vi "开机添加默认配置文件.vi"(8 "error in (no error)":errorcluster caption="错误输入（无错误）", 11 "恢复默认方式":enum16{"无配置开机恢复", "手动恢复"}(ring)) -> (0 "error out":errorcluster caption="错误输出")   [LabVIEW 2016, in "环境动力监测库.lvlib"]
uses:
  <vilib>/Utility/config.llb/NI_LVConfig.lvlib
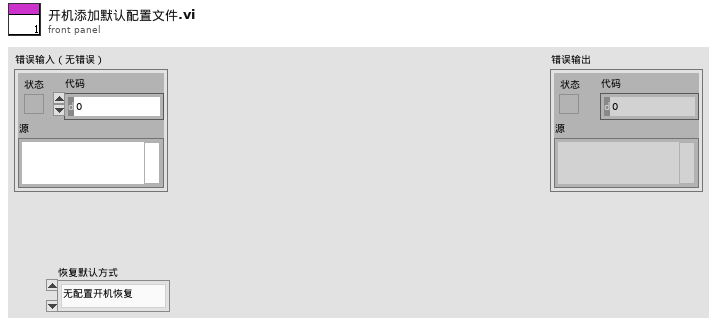
[diagram p1: front panel]
types:
  T1 = typedef "NI_LVConfig.lvlib/Config Data RefNum.ctl" = refnum<k1>
  T2 = cluster{"监测项描述:输出":string, "连接方式":enum16{"串口", "TCP"}, "端口":string, "IP address:":string, "Port:":string, "站号":u64, "传感器型号":string, "波特率":u64, "data bits":u64, "停止位":u16, "奇偶校验":u16}
  T3 = cluster{"监测项描述:输出":string, "端口":enum16{"AI0", "AI1", "AI2", "AI3", "AI4", "DI0", "DI1", "DI2", "DI3", "DI4", "DO0", "DO1", "DO2", "DO3", "DO4", "X0", "X1", "X2", "X3", "X4", "X5", "X6", "X7", "X8", "X9"}, "告警方式":enum32{"禁用告警", "闭合告警", "断开告警"}, "传感器型号":enum16{"PLC", "ZLAN"}}
  T4 = cluster{"监测项描述:输出":string, "端口":enum16{"AI0", "AI1", "AI2", "AI3", "AI4", "DI0", "DI1", "DI2", "DI3", "DI4", "DO0", "DO1", "DO2", "DO3", "DO4", "X0", "X1", "X2", "X3", "X4", "X5", "X6", "X7", "X8", "X9"}, "告警方式":enum32{"禁用告警", "闭合告警", "断开告警"}, "传感器型号":enum16{"PLC", "ZLAN"}, "声光告警启用":bool}
  T5 = cluster{"监测项描述:输出":string, "端口":enum16{"AI0", "AI1", "AI2", "AI3", "AI4", "DI0", "DI1", "DI2", "DI3", "DI4", "DO0", "DO1", "DO2", "DO3", "DO4", "X0", "X1", "X2", "X3", "X4", "X5", "X6", "X7", "X8", "X9"}, "告警方式":enum32{"禁用告警", "闭合告警", "断开告警"}, "传感器型号":enum16{"PLC", "ZLAN", "ART"}, "声光告警启用":bool}
  T6 = enum16{"AI0", "AI1", "AI2", "AI3", "AI4", "DI0", "DI1", "DI2", "DI3", "DI4", "DO0", "DO1", "DO2", "DO3", "DO4", "X0", "X1", "X2", "X3", "X4", "X5", "X6", "X7", "X8", "X9"}[]
  T7 = cluster{"漏水监测配置":cluster{"监测项描述:输出":string, "端口:":enum16{"AI0", "AI1", "AI2", "AI3", "AI4", "DI0", "DI1", "DI2", "DI3", "DI4", "DO0", "DO1", "DO2", "DO3", "DO4", "X0", "X1", "X2", "X3", "X4", "X5", "X6", "X7", "X8", "X9", "X10", "X11", "X12", "X13", "X14", "X15", "X16", "X17", "X18", "X19", "X20", "X21", "X22", "X23"}, "告警参数:":enum32{"禁用告警", "闭合告警", "断开告警"}, "传感器型号:":enum16{"PLC", "ZLAN", "ART"}, "声光告警启用":bool}, "门禁开关监测配置":cluster{"监测项描述:输出":string, "端口:":enum16{"AI0", "AI1", "AI2", "AI3", "AI4", "DI0", "DI1", "DI2", "DI3", "DI4", "DO0", "DO1", "DO2", "DO3", "DO4", "X0", "X1", "X2", "X3", "X4", "X5", "X6", "X7", "X8", "X9", "X10", "X11", "X12", "X13", "X14", "X15", "X16", "X17", "X18", "X19", "X20", "X21", "X22", "X23"}, "告警参数:":enum32{"禁用告警", "闭合告警", "断开告警"}, "传感器型号:":enum16{"PLC", "ZLAN", "ART"}, "声光告警启用":bool}, "门禁开关监测配置2":cluster{"监测项描述:输出":string, "端口:":enum16{"AI0", "AI1", "AI2", "AI3", "AI4", "DI0", "DI1", "DI2", "DI3", "DI4", "DO0", "DO1", "DO2", "DO3", "DO4", "X0", "X1", "X2", "X3", "X4", "X5", "X6", "X7", "X8", "X9", "X10", "X11", "X12", "X13", "X14", "X15", "X16", "X17", "X18", "X19", "X20", "X21", "X22", "X23"}, "告警参数:":enum32{"禁用告警", "闭合告警", "断开告警"}, "传感器型号:":enum16{"PLC", "ZLAN", "ART"}, "声光告警启用":bool}, "温湿度监测配置":cluster{"监测项描述:输出":string, "端口:":enum16{"AI0", "AI1", "AI2", "AI3", "AI4", "DI0", "DI1", "DI2", "DI3", "DI4", "DO0", "DO1", "DO2", "DO3", "DO4", "X0", "X1", "X2", "X3", "X4", "X5", "X6", "X7", "X8", "X9", "X10", "X11", "X12", "X13", "X14", "X15", "X16", "X17", "X18", "X19", "X20", "X21", "X22", "X23"}, "告警参数:":enum32{"禁用告警", "闭合告警", "断开告警"}, "传感器型号:":enum16{"PLC", "ZLAN", "ART"}, "声光告警启用":bool}, "烟雾监测配置":cluster{"监测项描述:输出":string, "端口:":enum16{"AI0", "AI1", "AI2", "AI3", "AI4", "DI0", "DI1", "DI2", "DI3", "DI4", "DO0", "DO1", "DO2", "DO3", "DO4", "X0", "X1", "X2", "X3", "X4", "X5", "X6", "X7", "X8", "X9", "X10", "X11", "X12", "X13", "X14", "X15", "X16", "X17", "X18", "X19", "X20", "X21", "X22", "X23"}, "告警参数:":enum32{"禁用告警", "闭合告警", "断开告警"}, "传感器型号:":enum16{"PLC", "ZLAN", "ART"}, "声光告警启用":bool}, "冰箱监测配置":cluster{"监测项描述:输出":string, "端口:":enum16{"AI0", "AI1", "AI2", "AI3", "AI4", "DI0", "DI1", "DI2", "DI3", "DI4", "DO0", "DO1", "DO2", "DO3", "DO4", "X0", "X1", "X2", "X3", "X4", "X5", "X6", "X7", "X8", "X9", "X10", "X11", "X12", "X13", "X14", "X15", "X16", "X17", "X18", "X19", "X20", "X21", "X22", "X23"}, "告警参数:":enum32{"禁用告警", "闭合告警", "断开告警"}, "传感器型号:":enum16{"PLC", "ZLAN", "ART"}, "声光告警启用":bool}, "排气扇监测配置":cluster{"监测项描述:输出":string, "端口:":enum16{"AI0", "AI1", "AI2", "AI3", "AI4", "DI0", "DI1", "DI2", "DI3", "DI4", "DO0", "DO1", "DO2", "DO3", "DO4", "X0", "X1", "X2", "X3", "X4", "X5", "X6", "X7", "X8", "X9", "X10", "X11", "X12", "X13", "X14", "X15", "X16", "X17", "X18", "X19", "X20", "X21", "X22", "X23"}, "告警参数:":enum32{"禁用告警", "闭合告警", "断开告警"}, "传感器型号:":enum16{"PLC", "ZLAN", "ART"}, "声光告警启用":bool}, "红外入侵监测配置":cluster{"监测项描述:输出":string, "端口:":enum16{"AI0", "AI1", "AI2", "AI3", "AI4", "DI0", "DI1", "DI2", "DI3", "DI4", "DO0", "DO1", "DO2", "DO3", "DO4", "X0", "X1", "X2", "X3", "X4", "X5", "X6", "X7", "X8", "X9", "X10", "X11", "X12", "X13", "X14", "X15", "X16", "X17", "X18", "X19", "X20", "X21", "X22", "X23"}, "告警参数:":enum32{"禁用告警", "闭合告警", "断开告警"}, "传感器型号:":enum16{"PLC", "ZLAN", "ART"}, "声光告警启用":bool}, "振动监测配置":cluster{"监测项描述:输出":string, "端口:":enum16{"AI0", "AI1", "AI2", "AI3", "AI4", "DI0", "DI1", "DI2", "DI3", "DI4", "DO0", "DO1", "DO2", "DO3", "DO4", "X0", "X1", "X2", "X3", "X4", "X5", "X6", "X7", "X8", "X9", "X10", "X11", "X12", "X13", "X14", "X15", "X16", "X17", "X18", "X19", "X20", "X21", "X22", "X23"}, "告警参数:":enum32{"禁用告警", "闭合告警", "断开告警"}, "传感器型号:":enum16{"PLC", "ZLAN", "ART"}, "声光告警启用":bool}}
  T8 = cluster{"市电监测":bool, "用水量监测":bool, "烟雾监测":bool, "温度湿度":bool, "振动监测":bool, "红外入侵监测":bool, "漏水监测":bool, "门禁开关监测":bool, "门禁开关监测2":bool, "视频监测":bool, "UPS监测":bool, "空调监测":bool, "冰箱监测":bool, "排气扇监测":bool, "蓄电池监测":bool, "蓄电池监测2":bool, "GPS监测":bool, "北斗监测":bool, "气象监测":bool, "智能门禁监测":bool}
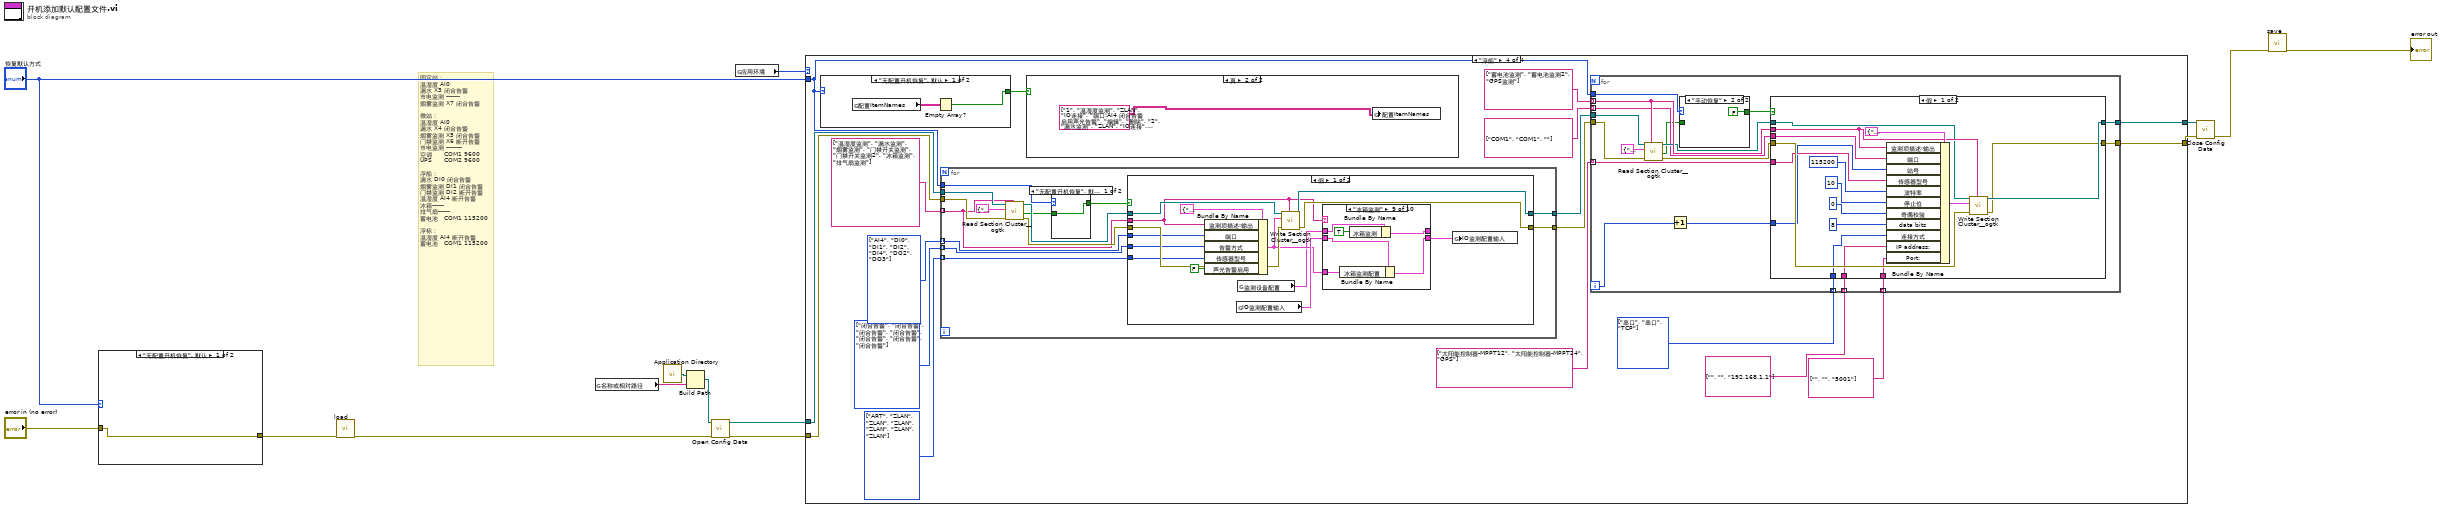
[diagram p0: block diagram]
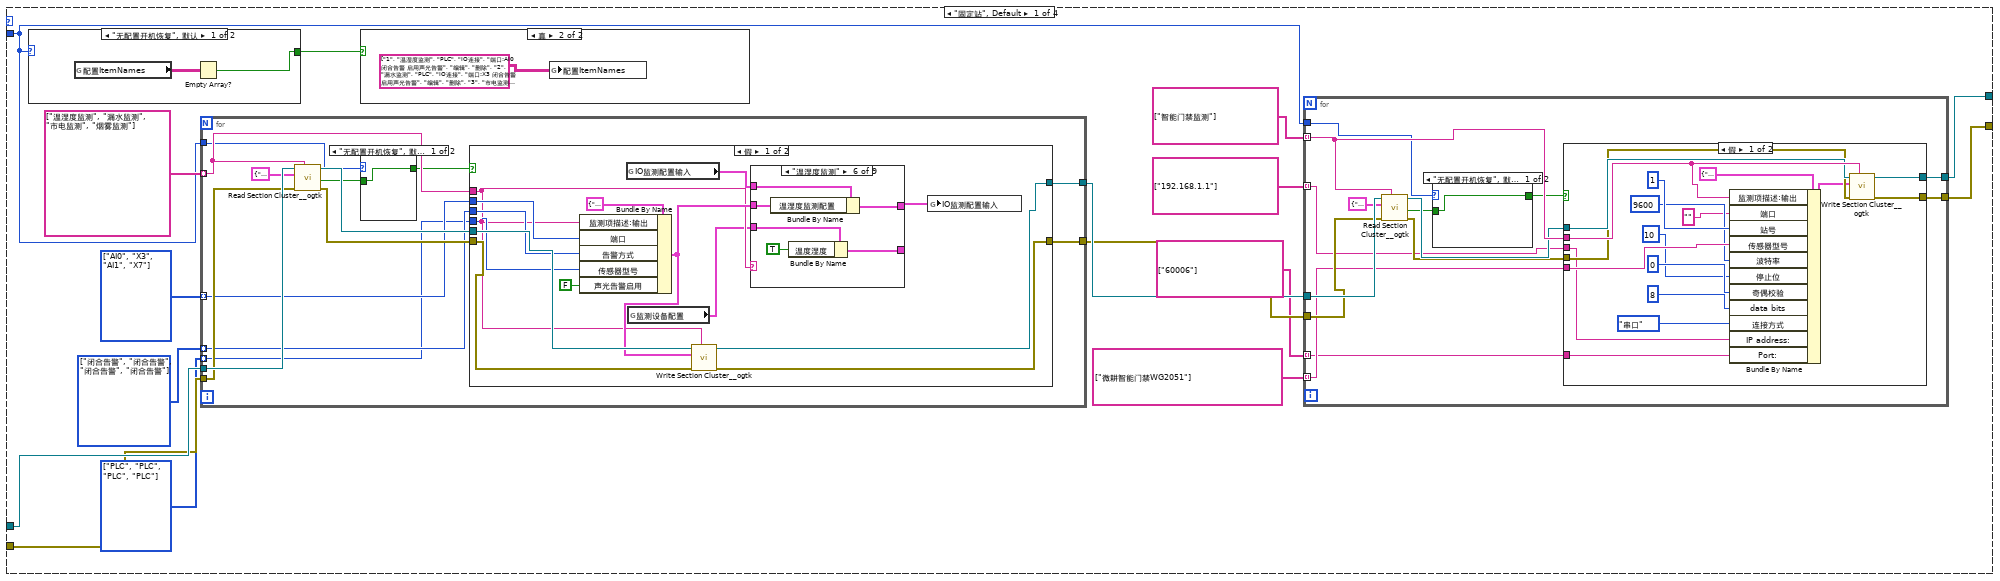
[diagram p3: hidden frame]
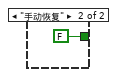
[diagram p4: hidden frame]
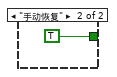
[diagram p6: hidden frame]
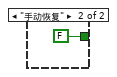
[diagram p8: hidden frame]
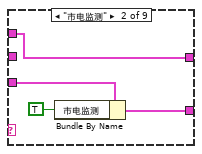
[diagram p10: hidden frame]
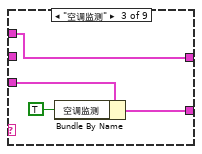
[diagram p11: hidden frame]
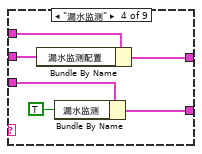
[diagram p12: hidden frame]
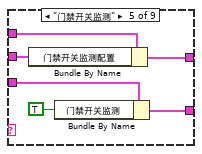
[diagram p13: hidden frame]
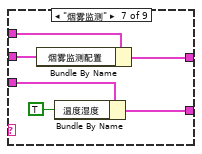
[diagram p14: hidden frame]
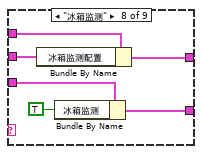
[diagram p15: hidden frame]
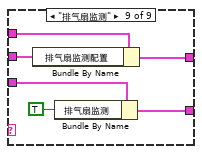
[diagram p16: hidden frame]
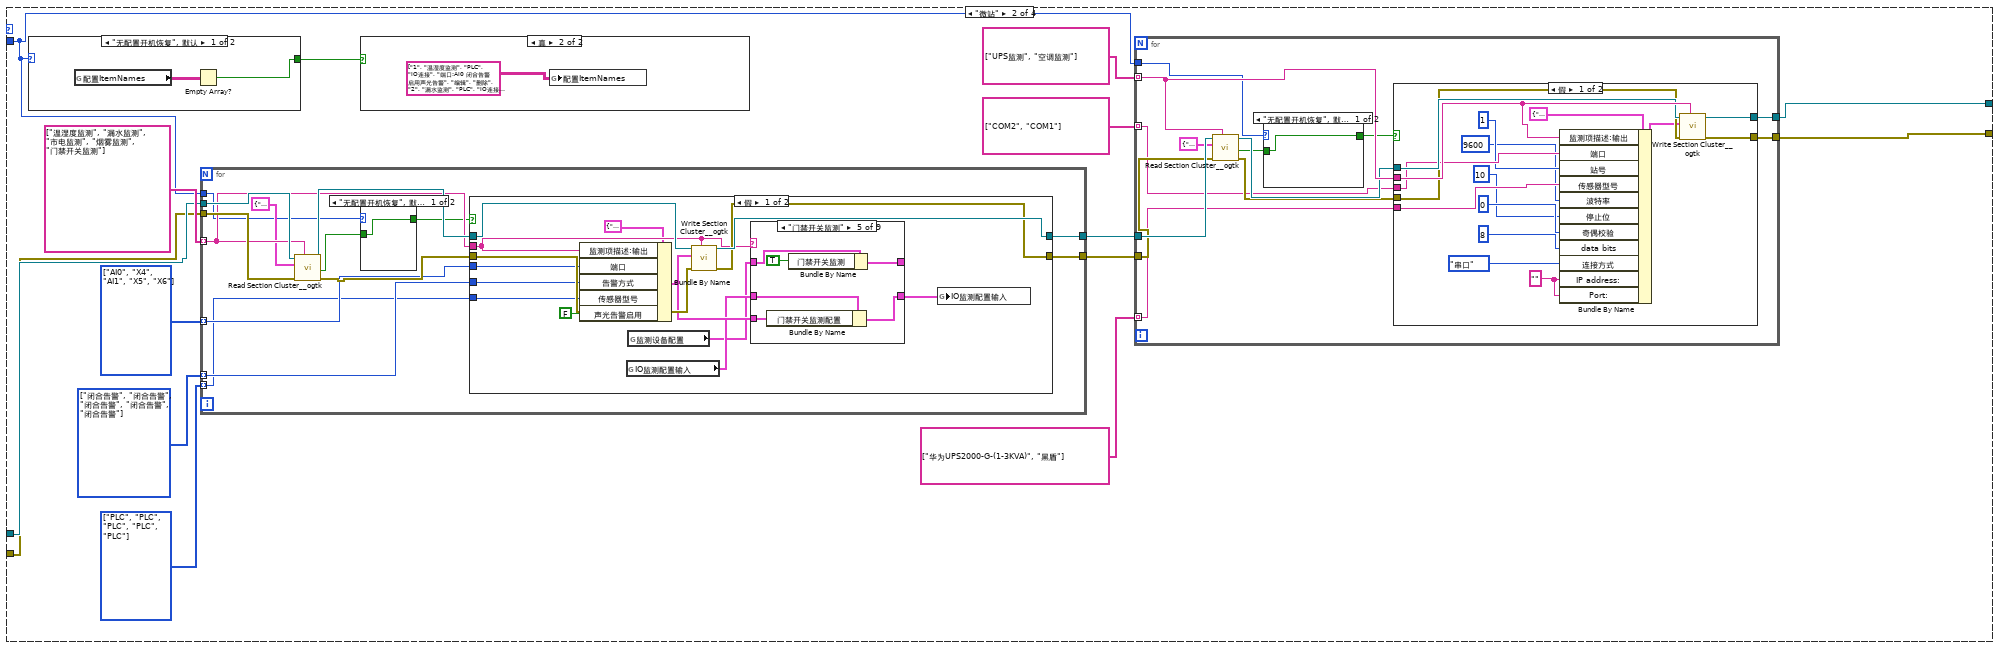
[diagram p18: hidden frame]
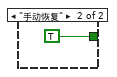
[diagram p19: hidden frame]
diagram:
  # "固定站：\n温湿度 AI0\n漏水 X3 闭合告警\n市电监测 -------\n烟雾监测 X7 闭合告警\n\n微站：\n温湿度 AI0\n漏水 X4 闭合告警\n烟雾监测 X5 闭合告警\n门禁监测 X6 断开告警\n市电监测 --------\n空调      COM1 9600\nUPS      COM2 9600\n\n浮船：\n漏水 DI0 闭合告警\n烟雾监测 DI1 闭合告警\n门禁监测 DI2 断开告警\n温湿度 AI4 断开告警\n冰箱------\n排气扇------\n蓄电池   COM1 115200\n\n浮标：\n温湿度 AI4 断开告警\n蓄电池   COM1 115200"
  n1 = case shown="\"无配置开机恢复\", 默认" "恢复默认方式" {
    tunnel: "error in (no error)" -> [w15 w16]
    tunnel: [w15 w16] -> w3
    frame "无配置开机恢复", Default {
    }
    frame "手动恢复" {
    }
  }
  n2 = call "load.vi"("error in (no error)"=w3) -> ("error out"=w7:errorcluster)  [unwired: 10 in]
  n3 = global read "内部交互全局变量.vi" "名称或相对路径"() -> (w4:string)
  n4 = call <vilib>:"Application Directory.vi"() -> ("Application Directory"=w13:path)
  n5 = Build Path(base path=w13, name or relative path=w4) -> (appended path=w12:path)
  n6 = call <vilib>:"Open Config Data.vi"("error in (no error)"=w7, "configuration file path"=w12) -> ("error out"=w10:errorcluster, "refnum"=w11:T1)  [unwired: 7 in, 1 out]
  n7 = global read "外部交互全局变量.vi" "应用环境"() -> (w14:enum16{"固定站", "微站", "浮标", "浮船"})
  n8 = case shown="\"浮船\"" w14 {
    tunnel: w11 -> [w31 w163 w293 w426]
    tunnel: w10 -> [w30 w162 w292 w425]
    tunnel: [w19 w158 w288 w421] -> w9
    tunnel: [w18 w157 w287 w420] -> w8
    tunnel: "恢复默认方式" -> [w20 w150 w280 w413]
    frame "固定站", Default {
      w27 = enum16{"PLC", "ZLAN"}[] [enum."PLC", enum."PLC", enum."PLC", enum."PLC"] items=["PLC", "ZLAN"]
      w28 = enum32{"禁用告警", "闭合告警", "断开告警"}[] [enum."闭合告警", enum."闭合告警", enum."闭合告警", enum."闭合告警"] items=["禁用告警", "闭合告警", "断开告警"]
      w29 = T6 [enum."AI0", enum."X3", enum."AI1", enum."X7"] items=["AI0", "AI1", "AI2", "AI3", "AI4", "DI0", "DI1", "DI2", "DI3", "DI4", "DO0", "DO1", "DO2", "DO3", "DO4", "X0", "X1", "X2", "X3", "X4", "X5", "X6", "X7", "X8", "X9"]
      n9 = case shown="\"无配置开机恢复\", 默认" w20 {
        tunnel: [w68 TRUE ("empty?")] -> w26
        frame "无配置开机恢复", Default {
          n10 = global read "断电保存全局变量.vi" "配置ItemNames"() -> (w69:string[][])
          n11 = Empty Array?(array=w69) -> (empty?=w68:bool)
        }
        frame "手动恢复" {
        }
      }
      n12 = for {
        tunnel: string[] ["温湿度监测", "漏水监测", "市电监测", "烟雾监测"] -> [w81] mode=indexing
        tunnel: w31 -> [w85]
        tunnel: w30 -> [w84]
        tunnel: w29 -> [w80] mode=indexing
        tunnel: w28 -> [w79] mode=indexing
        tunnel: w27 -> [w78] mode=indexing
        tunnel: [w77] -> w22
        tunnel: [w76] -> w21
        tunnel: w20 -> [w72]
        n13 = call <userlib>:"Read Section Cluster__ogtk.vi"("section (optional)"=w81, "error in (no error)"=w84, "Section Formatted Cluster Type"=T3 {"监测项描述:输出"="烟雾监测", "端口"=enum."X8", "告警方式"=enum."闭合告警", "传感器型号"=enum."PLC"} ("簇1输入"), "refnum"=w85) -> ("error out"=w82:errorcluster, "all found?"=w74:bool, "dup refnum"=w83:T1)  [unwired: 3 in, 2 out]
        n14 = case shown="\"无配置开机恢复\", 默认" w72 {
          tunnel: [w86 FALSE] -> w73
          tunnel: w74 -> [w86 _]
          frame "无配置开机恢复", Default {
          }
          frame "手动恢复" {
          }
        }
        n15 = case shown="假" w73 {
          tunnel: w83 -> [w101 w149]
          tunnel: w82 -> [w100 w148]
          tunnel: w81 -> [w92 _]
          tunnel: w80 -> [w99 _]
          tunnel: w79 -> [w94 _]
          tunnel: w78 -> [w98 _]
          tunnel: [w97 w149] -> w77
          tunnel: [w96 w148] -> w76
          frame False {
            n16 = Bundle By Name(cluster=T4 {"监测项描述:输出"="", "端口"=enum."AI0", "告警方式"=enum."禁用告警", "传感器型号"=enum."PLC", "声光告警启用"=FALSE} ("簇1输出"), "监测项描述:输出"=w92, "端口"=w99, "告警方式"=w94, "传感器型号"=w98, "声光告警启用"=FALSE) -> (w93:T4)
            n17 = global read "断电保存全局变量.vi" "IO监测配置输入"() -> (w95:T7)
            n18 = global read "断电保存全局变量.vi" "监测设备配置"() -> (w91:T8)
            n19 = call <userlib>:"Write Section Cluster__ogtk.vi"("section (optional)"=w92, "error in (no error)"=w100, "Section Formatted Cluster"=w93, "refnum"=w101) -> ("error out"=w96:errorcluster, "dup refnum"=w97:T1)  [unwired: 6 in]
            n20 = case shown="\"温湿度监测\"" w92 {
              tunnel: w95 -> [w103 w107 w111 w117 w123 w129 w135 w141 w147]
              tunnel: [w103 w107 w111 w116 w122 w128 w134 w140 w146] -> w90
              tunnel: w93 -> [_ _ _ w115 w121 w127 w133 w139 w145]
              tunnel: w91 -> [w102 w106 w110 w114 w119 w126 w132 w138 w144]
              tunnel: [w102 w104 w109 w113 w120 w125 w131 w137 w143] -> _
              frame "假", Default {
              }
              frame "市电监测" {
                n21 = Bundle By Name(cluster=w106, "市电监测"=TRUE) -> (w104:T8)
              }
              frame "空调监测" {
                n22 = Bundle By Name(cluster=w110, "空调监测"=TRUE) -> (w109:T8)
              }
              frame "漏水监测" {
                n23 = Bundle By Name(cluster=w117, "漏水监测配置"=w115) -> (w116:T7)
                n24 = Bundle By Name(cluster=w114, "漏水监测"=TRUE) -> (w113:T8)
              }
              frame "门禁开关监测" {
                n25 = Bundle By Name(cluster=w123, "门禁开关监测配置"=w121) -> (w122:T7)
                n26 = Bundle By Name(cluster=w119, "门禁开关监测"=TRUE) -> (w120:T8)
              }
              frame "温湿度监测" {
                n27 = Bundle By Name(cluster=w129, "温湿度监测配置"=w127) -> (w128:T7)
                n28 = Bundle By Name(cluster=w126, "温度湿度"=TRUE) -> (w125:T8)
              }
              frame "烟雾监测" {
                n29 = Bundle By Name(cluster=w135, "烟雾监测配置"=w133) -> (w134:T7)
                n30 = Bundle By Name(cluster=w132, "温度湿度"=TRUE) -> (w131:T8)
              }
              frame "冰箱监测" {
                n31 = Bundle By Name(cluster=w141, "冰箱监测配置"=w139) -> (w140:T7)
                n32 = Bundle By Name(cluster=w138, "冰箱监测"=TRUE ("市电监测")) -> (w137:T8)
              }
              frame "排气扇监测" {
                n33 = Bundle By Name(cluster=w147, "排气扇监测配置"=w145) -> (w146:T7)
                n34 = Bundle By Name(cluster=w144, "排气扇监测"=TRUE) -> (w143:T8)
              }
            }
            n35 = global write "断电保存全局变量.vi" "IO监测配置输入"(w90) -> ()
          }
          frame True {
          }
        }
      }
      n36 = case shown="真" w26 {
        frame False {
        }
        frame True {
          n37 = global write "断电保存全局变量.vi" "配置ItemNames"(string[][] [["1", "温湿度监测", "PLC", "IO连接", "端口:AI0 闭合告警 启用声光告警", "编辑", "删除"], ["2", "漏水监测", "PLC", "IO连接", "端口:X3 闭合告警 启用声光告警", "编辑", "删除"], ["3", "市电监测", "PLC", "IO连接", "端口:AI1 闭合告警 启用声光告警", "编辑", "删除"], ["4", "烟雾监测", "PLC", "IO连接", "端口:X7 闭合告警 启用声光告警", "编辑", "删除"], ["5", "智能门禁监测", "微耕智能门禁WG2051", "TCP连接", "IP:127.0.0.1 Port:60006 不启用声光告警", "编辑", "删除"]] ("配置ItemNames")) -> ()
        }
      }
      n38 = for {
        tunnel: w22 -> [w46]
        tunnel: w21 -> [w45]
        tunnel: string[] ["智能门禁监测"] -> [w44] mode=indexing
        tunnel: [w41] -> w19
        tunnel: [w40] -> w18
        tunnel: string[] ["192.168.1.1"] -> [w39] mode=indexing
        tunnel: string[] ["微耕智能门禁WG2051"] -> [w38] mode=indexing
        tunnel: w20 -> [w36]
        tunnel: string[] ["60006"] -> [w33] mode=indexing
        n39 = call <userlib>:"Read Section Cluster__ogtk.vi"("section (optional)"=w44, "error in (no error)"=w45, "Section Formatted Cluster Type"=T2 {"监测项描述:输出"="", "连接方式"=enum."串口", "端口"="", "IP address:"="", "Port:"="", "站号"=19200, "传感器型号"="", "波特率"=19200, "data bits"=8, "停止位"=10, "奇偶校验"=0} ("输出簇"), "refnum"=w46) -> ("error out"=w42:errorcluster, "all found?"=w35:bool, "dup refnum"=w43:T1)  [unwired: 3 in, 2 out]
        n40 = case shown="\"无配置开机恢复\", 默认" w36 {
          tunnel: [w47 FALSE] -> w34
          tunnel: w35 -> [w47 _]
          frame "无配置开机恢复", Default {
          }
          frame "手动恢复" {
          }
        }
        n41 = case shown="假" w34 {
          tunnel: w44 -> [w64 _]
          tunnel: w43 -> [w63 w67]
          tunnel: w42 -> [w62 w66]
          tunnel: [w60 w67] -> w41
          tunnel: [w59 w66] -> w40
          tunnel: w39 -> [w50 _]
          tunnel: w38 -> [w57 _]
          tunnel: w33 -> [w49 _]
          frame False {
            n42 = Bundle By Name(cluster=T2 {"监测项描述:输出"="", "连接方式"=enum."串口", "端口"="", "IP address:"="", "Port:"="", "站号"=19200, "传感器型号"="", "波特率"=19200, "data bits"=8, "停止位"=10, "奇偶校验"=0} ("输出簇"), "监测项描述:输出"=w64, "端口"="" ("IP address:"), "站号"=u64 1, "传感器型号"=w57, "波特率"=u64 9600, "停止位"=u16 10, "奇偶校验"=u16 0, "data bits"=u64 8, "连接方式"=enum16{"串口", "TCP"}."串口", "IP address:"=w50, "Port:"=w49) -> (w61:T2)
            n43 = call <userlib>:"Write Section Cluster__ogtk.vi"("section (optional)"=w64, "error in (no error)"=w62, "Section Formatted Cluster"=w61, "refnum"=w63) -> ("error out"=w59:errorcluster, "dup refnum"=w60:T1)  [unwired: 6 in]
          }
          frame True {
          }
        }
      }
    }
    frame "微站" {
      w152 = enum16{"PLC", "ZLAN"}[] [enum."PLC", enum."PLC", enum."PLC", enum."PLC", enum."PLC"] items=["PLC", "ZLAN"]
      w153 = enum32{"禁用告警", "闭合告警", "断开告警"}[] [enum."闭合告警", enum."闭合告警", enum."闭合告警", enum."闭合告警", enum."闭合告警"] items=["禁用告警", "闭合告警", "断开告警"]
      w154 = T6 [enum."AI0", enum."X4", enum."AI1", enum."X5", enum."X6"] items=["AI0", "AI1", "AI2", "AI3", "AI4", "DI0", "DI1", "DI2", "DI3", "DI4", "DO0", "DO1", "DO2", "DO3", "DO4", "X0", "X1", "X2", "X3", "X4", "X5", "X6", "X7", "X8", "X9"]
      n44 = case shown="\"无配置开机恢复\", 默认" w150 {
        tunnel: [w165 TRUE ("empty?")] -> w151
        frame "无配置开机恢复", Default {
          n45 = global read "断电保存全局变量.vi" "配置ItemNames"() -> (w166:string[][])
          n46 = Empty Array?(array=w166) -> (empty?=w165:bool)
        }
        frame "手动恢复" {
        }
      }
      n47 = for {
        tunnel: string[] ["温湿度监测", "漏水监测", "市电监测", "烟雾监测", "门禁开关监测"] -> [w211] mode=indexing
        tunnel: w163 -> [w215]
        tunnel: w162 -> [w214]
        tunnel: w154 -> [w210] mode=indexing
        tunnel: w153 -> [w209] mode=indexing
        tunnel: w152 -> [w208] mode=indexing
        tunnel: [w207] -> w161
        tunnel: [w206] -> w160
        tunnel: w150 -> [w204]
        n48 = call <userlib>:"Read Section Cluster__ogtk.vi"("section (optional)"=w211, "error in (no error)"=w214, "Section Formatted Cluster Type"=T3 {"监测项描述:输出"="烟雾监测", "端口"=enum."X8", "告警方式"=enum."闭合告警", "传感器型号"=enum."PLC"} ("簇1输入"), "refnum"=w215) -> ("error out"=w212:errorcluster, "all found?"=w203:bool, "dup refnum"=w213:T1)  [unwired: 3 in, 2 out]
        n49 = case shown="\"无配置开机恢复\", 默认" w204 {
          tunnel: [w216 FALSE] -> w202
          tunnel: w203 -> [w216 _]
          frame "无配置开机恢复", Default {
          }
          frame "手动恢复" {
          }
        }
        n50 = case shown="假" w202 {
          tunnel: w213 -> [w231 w279]
          tunnel: w212 -> [w230 w278]
          tunnel: w211 -> [w224 _]
          tunnel: w210 -> [w229 _]
          tunnel: w209 -> [w228 _]
          tunnel: w208 -> [w227 _]
          tunnel: [w226 w279] -> w207
          tunnel: [w225 w278] -> w206
          frame False {
            n51 = Bundle By Name(cluster=T4 {"监测项描述:输出"="", "端口"=enum."AI0", "告警方式"=enum."禁用告警", "传感器型号"=enum."PLC", "声光告警启用"=FALSE} ("簇1输出"), "监测项描述:输出"=w224, "端口"=w229, "告警方式"=w228, "传感器型号"=w227, "声光告警启用"=FALSE) -> (w223:T4)
            n52 = global read "断电保存全局变量.vi" "IO监测配置输入"() -> (w222:T7)
            n53 = global read "断电保存全局变量.vi" "监测设备配置"() -> (w220:T8)
            n54 = call <userlib>:"Write Section Cluster__ogtk.vi"("section (optional)"=w224, "error in (no error)"=w230, "Section Formatted Cluster"=w223, "refnum"=w231) -> ("error out"=w225:errorcluster, "dup refnum"=w226:T1)  [unwired: 6 in]
            n55 = case shown="\"门禁开关监测\"" w224 {
              tunnel: w222 -> [w233 w237 w241 w247 w253 w259 w265 w271 w277]
              tunnel: [w233 w237 w241 w246 w252 w258 w264 w270 w276] -> w221
              tunnel: w223 -> [_ _ _ w245 w251 w257 w263 w269 w275]
              tunnel: w220 -> [w232 w236 w240 w244 w249 w256 w262 w268 w274]
              tunnel: [w232 w234 w239 w243 w250 w255 w261 w267 w273] -> _
              frame "假", Default {
              }
              frame "市电监测" {
                n56 = Bundle By Name(cluster=w236, "市电监测"=TRUE) -> (w234:T8)
              }
              frame "空调监测" {
                n57 = Bundle By Name(cluster=w240, "空调监测"=TRUE) -> (w239:T8)
              }
              frame "漏水监测" {
                n58 = Bundle By Name(cluster=w247, "漏水监测配置"=w245) -> (w246:T7)
                n59 = Bundle By Name(cluster=w244, "漏水监测"=TRUE) -> (w243:T8)
              }
              frame "门禁开关监测" {
                n60 = Bundle By Name(cluster=w253, "门禁开关监测配置"=w251) -> (w252:T7)
                n61 = Bundle By Name(cluster=w249, "门禁开关监测"=TRUE) -> (w250:T8)
              }
              frame "温湿度监测" {
                n62 = Bundle By Name(cluster=w259, "温湿度监测配置"=w257) -> (w258:T7)
                n63 = Bundle By Name(cluster=w256, "温度湿度"=TRUE) -> (w255:T8)
              }
              frame "烟雾监测" {
                n64 = Bundle By Name(cluster=w265, "烟雾监测配置"=w263) -> (w264:T7)
                n65 = Bundle By Name(cluster=w262, "温度湿度"=TRUE) -> (w261:T8)
              }
              frame "冰箱监测" {
                n66 = Bundle By Name(cluster=w271, "冰箱监测配置"=w269) -> (w270:T7)
                n67 = Bundle By Name(cluster=w268, "冰箱监测"=TRUE ("市电监测")) -> (w267:T8)
              }
              frame "排气扇监测" {
                n68 = Bundle By Name(cluster=w277, "排气扇监测配置"=w275) -> (w276:T7)
                n69 = Bundle By Name(cluster=w274, "排气扇监测"=TRUE) -> (w273:T8)
              }
            }
            n70 = global write "断电保存全局变量.vi" "IO监测配置输入"(w221) -> ()
          }
          frame True {
          }
        }
      }
      n71 = case shown="真" w151 {
        frame False {
        }
        frame True {
          n72 = global write "断电保存全局变量.vi" "配置ItemNames"(string[][] [["1", "温湿度监测", "PLC", "IO连接", "端口:AI0 闭合告警 启用声光告警", "编辑", "删除"], ["2", "漏水监测", "PLC", "IO连接", "端口:X4 闭合告警 启用声光告警", "编辑", "删除"], ["3", "市电监测", "PLC", "IO连接", "端口:AI1 闭合告警 启用声光告警", "编辑", "删除"], ["4", "烟雾监测", "PLC", "IO连接", "端口:X5 闭合告警 启用声光告警", "编辑", "删除"], ["5", "门禁开关监测", "PLC", "IO连接", "端口:X6 闭合告警 启用声光告警", "编辑", "删除"], ["6", "UPS监测", "华为UPS2000-G-(1-3KVA)", "串口连接", "端口:COM2 站号:1 波特率:9600", "编辑", "删除"], ["7", "空调监测", "黑盾", "串口连接", "串口:COM1 站号:1 波特率:9600", "编辑", "删除"]] ("配置ItemNames")) -> ()
        }
      }
      n73 = for {
        tunnel: w161 -> [w181]
        tunnel: w160 -> [w180]
        tunnel: string[] ["UPS监测", "空调监测"] -> [w179] mode=indexing
        tunnel: [w176] -> w158
        tunnel: [w175] -> w157
        tunnel: string[] ["COM2", "COM1"] -> [w174] mode=indexing
        tunnel: string[] ["华为UPS2000-G-(1-3KVA)", "黑盾"] -> [w173] mode=indexing
        tunnel: w150 -> [w171]
        n74 = call <userlib>:"Read Section Cluster__ogtk.vi"("section (optional)"=w179, "error in (no error)"=w180, "Section Formatted Cluster Type"=T2 {"监测项描述:输出"="", "连接方式"=enum."串口", "端口"="", "IP address:"="", "Port:"="", "站号"=19200, "传感器型号"="", "波特率"=19200, "data bits"=8, "停止位"=10, "奇偶校验"=0} ("输出簇"), "refnum"=w181) -> ("error out"=w177:errorcluster, "all found?"=w170:bool, "dup refnum"=w178:T1)  [unwired: 3 in, 2 out]
        n75 = case shown="\"无配置开机恢复\", 默认" w171 {
          tunnel: [w182 FALSE] -> w169
          tunnel: w170 -> [w182 _]
          frame "无配置开机恢复", Default {
          }
          frame "手动恢复" {
          }
        }
        n76 = case shown="假" w169 {
          tunnel: w179 -> [w198 _]
          tunnel: w178 -> [w197 w201]
          tunnel: w177 -> [w196 w200]
          tunnel: [w194 w201] -> w176
          tunnel: [w193 w200] -> w175
          tunnel: w174 -> [w192 _]
          tunnel: w173 -> [w190 _]
          frame False {
            w184 = "" ("IP address:")
            n77 = Bundle By Name(cluster=T2 {"监测项描述:输出"="", "连接方式"=enum."串口", "端口"="", "IP address:"="", "Port:"="", "站号"=19200, "传感器型号"="", "波特率"=19200, "data bits"=8, "停止位"=10, "奇偶校验"=0} ("输出簇"), "监测项描述:输出"=w198, "端口"=w192, "站号"=u64 1, "传感器型号"=w190, "波特率"=u64 9600, "停止位"=u16 10, "奇偶校验"=u16 0, "data bits"=u64 8, "连接方式"=enum16{"串口", "TCP"}."串口", "IP address:"=w184, "Port:"=w184) -> (w195:T2)
            n78 = call <userlib>:"Write Section Cluster__ogtk.vi"("section (optional)"=w198, "error in (no error)"=w196, "Section Formatted Cluster"=w195, "refnum"=w197) -> ("error out"=w193:errorcluster, "dup refnum"=w194:T1)  [unwired: 6 in]
          }
          frame True {
          }
        }
      }
    }
    frame "浮标" {
      w282 = enum16{"PLC", "ZLAN", "ART"}[] [enum."ART"] items=["PLC", "ZLAN", "ART"]
      w283 = enum32{"禁用告警", "闭合告警", "断开告警"}[] [enum."闭合告警"] items=["禁用告警", "闭合告警", "断开告警"]
      w284 = T6 [enum."AI1"] items=["AI0", "AI1", "AI2", "AI3", "AI4", "DI0", "DI1", "DI2", "DI3", "DI4", "DO0", "DO1", "DO2", "DO3", "DO4", "X0", "X1", "X2", "X3", "X4", "X5", "X6", "X7", "X8", "X9"]
      n79 = case shown="\"无配置开机恢复\", 默认" w280 {
        tunnel: [w295 TRUE ("empty?")] -> w281
        frame "无配置开机恢复", Default {
          n80 = global read "断电保存全局变量.vi" "配置ItemNames"() -> (w296:string[][])
          n81 = Empty Array?(array=w296) -> (empty?=w295:bool)
        }
        frame "手动恢复" {
        }
      }
      n82 = for {
        tunnel: string[] ["温湿度监测"] -> [w341] mode=indexing
        tunnel: w293 -> [w345]
        tunnel: w292 -> [w344]
        tunnel: w284 -> [w340] mode=indexing
        tunnel: w283 -> [w339] mode=indexing
        tunnel: w282 -> [w338] mode=indexing
        tunnel: [w337] -> w291
        tunnel: [w336] -> w290
        tunnel: w280 -> [w332]
        n83 = call <userlib>:"Read Section Cluster__ogtk.vi"("section (optional)"=w341, "error in (no error)"=w344, "Section Formatted Cluster Type"=T3 {"监测项描述:输出"="烟雾监测", "端口"=enum."X8", "告警方式"=enum."闭合告警", "传感器型号"=enum."PLC"} ("簇1输入"), "refnum"=w345) -> ("error out"=w342:errorcluster, "all found?"=w334:bool, "dup refnum"=w343:T1)  [unwired: 3 in, 2 out]
        n84 = case shown="\"无配置开机恢复\", 默认" w332 {
          tunnel: [w346 FALSE] -> w333
          tunnel: w334 -> [w346 _]
          frame "无配置开机恢复", Default {
          }
          frame "手动恢复" {
          }
        }
        n85 = case shown="假" w333 {
          tunnel: w343 -> [w361 w409]
          tunnel: w342 -> [w360 w408]
          tunnel: w341 -> [w351 _]
          tunnel: w340 -> [w359 _]
          tunnel: w339 -> [w358 _]
          tunnel: w338 -> [w357 _]
          tunnel: [w356 w409] -> w337
          tunnel: [w355 w408] -> w336
          frame False {
            n86 = Bundle By Name(cluster=T5 {"监测项描述:输出"="", "端口"=enum."AI0", "告警方式"=enum."禁用告警", "传感器型号"=enum."PLC", "声光告警启用"=FALSE} ("簇1输出"), "监测项描述:输出"=w351, "端口"=w359, "告警方式"=w358, "传感器型号"=w357, "声光告警启用"=FALSE) -> (w352:T5)
            n87 = global read "断电保存全局变量.vi" "IO监测配置输入"() -> (w354:T7)
            n88 = global read "断电保存全局变量.vi" "监测设备配置"() -> (w350:T8)
            n89 = call <userlib>:"Write Section Cluster__ogtk.vi"("section (optional)"=w351, "error in (no error)"=w360, "Section Formatted Cluster"=w352, "refnum"=w361) -> ("error out"=w355:errorcluster, "dup refnum"=w356:T1)  [unwired: 6 in]
            n90 = case shown="\"温湿度监测\"" w351 {
              tunnel: w354 -> [w363 w367 w371 w377 w383 w389 w395 w401 w407]
              tunnel: [w363 w367 w371 w376 w382 w388 w394 w400 w406] -> w353
              tunnel: w352 -> [_ _ _ w375 w381 w387 w393 w399 w405]
              tunnel: w350 -> [w362 w366 w370 w374 w379 w386 w392 w398 w404]
              tunnel: [w362 w364 w369 w373 w380 w385 w391 w397 w403] -> _
              frame "假", Default {
              }
              frame "市电监测" {
                n91 = Bundle By Name(cluster=w366, "市电监测"=TRUE) -> (w364:T8)
              }
              frame "空调监测" {
                n92 = Bundle By Name(cluster=w370, "空调监测"=TRUE) -> (w369:T8)
              }
              frame "漏水监测" {
                n93 = Bundle By Name(cluster=w377, "漏水监测配置"=w375) -> (w376:T7)
                n94 = Bundle By Name(cluster=w374, "漏水监测"=TRUE) -> (w373:T8)
              }
              frame "门禁开关监测" {
                n95 = Bundle By Name(cluster=w383, "门禁开关监测配置"=w381) -> (w382:T7)
                n96 = Bundle By Name(cluster=w379, "门禁开关监测"=TRUE) -> (w380:T8)
              }
              frame "温湿度监测" {
                n97 = Bundle By Name(cluster=w389, "温湿度监测配置"=w387) -> (w388:T7)
                n98 = Bundle By Name(cluster=w386, "温度湿度"=TRUE) -> (w385:T8)
              }
              frame "烟雾监测" {
                n99 = Bundle By Name(cluster=w395, "烟雾监测配置"=w393) -> (w394:T7)
                n100 = Bundle By Name(cluster=w392, "温度湿度"=TRUE) -> (w391:T8)
              }
              frame "冰箱监测" {
                n101 = Bundle By Name(cluster=w401, "冰箱监测配置"=w399) -> (w400:T7)
                n102 = Bundle By Name(cluster=w398, "冰箱监测"=TRUE ("市电监测")) -> (w397:T8)
              }
              frame "排气扇监测" {
                n103 = Bundle By Name(cluster=w407, "排气扇监测配置"=w405) -> (w406:T7)
                n104 = Bundle By Name(cluster=w404, "排气扇监测"=TRUE) -> (w403:T8)
              }
            }
            n105 = global write "断电保存全局变量.vi" "IO监测配置输入"(w353) -> ()
          }
          frame True {
          }
        }
      }
      n106 = case shown="真" w281 {
        frame False {
        }
        frame True {
          n107 = global write "断电保存全局变量.vi" "配置ItemNames"(string[][] [["1", "温湿度监测", "ART", "IO连接", "端口:AI1 闭合告警 启用声光告警", "编辑", "删除"], ["2", "蓄电池监测", "太阳能控制器-MPPT12", "串口连接", "端口:COM8 站号:1 波特率:115200", "编辑", "删除"]] ("配置ItemNames")) -> ()
        }
      }
      n108 = for {
        tunnel: w291 -> [w311]
        tunnel: w290 -> [w310]
        tunnel: string[] ["蓄电池监测"] -> [w309] mode=indexing
        tunnel: [w306] -> w288
        tunnel: [w305] -> w287
        tunnel: string[] ["COM1"] -> [w304] mode=indexing
        tunnel: string[] ["太阳能控制器-MPPT12"] -> [w303] mode=indexing
        tunnel: w280 -> [w299]
        n109 = call <userlib>:"Read Section Cluster__ogtk.vi"("section (optional)"=w309, "error in (no error)"=w310, "Section Formatted Cluster Type"=T2 {"监测项描述:输出"="", "连接方式"=enum."串口", "端口"="", "IP address:"="", "Port:"="", "站号"=19200, "传感器型号"="", "波特率"=19200, "data bits"=8, "停止位"=10, "奇偶校验"=0} ("输出簇"), "refnum"=w311) -> ("error out"=w307:errorcluster, "all found?"=w301:bool, "dup refnum"=w308:T1)  [unwired: 3 in, 2 out]
        n110 = case shown="\"无配置开机恢复\", 默认" w299 {
          tunnel: [w312 FALSE] -> w300
          tunnel: w301 -> [w312 _]
          frame "无配置开机恢复", Default {
          }
          frame "手动恢复" {
          }
        }
        n111 = case shown="假" w300 {
          tunnel: w309 -> [w328 _]
          tunnel: w308 -> [w327 w331]
          tunnel: w307 -> [w326 w330]
          tunnel: [w324 w331] -> w306
          tunnel: [w323 w330] -> w305
          tunnel: w304 -> [w322 _]
          tunnel: w303 -> [w320 _]
          frame False {
            w314 = "" ("IP address:")
            n112 = Bundle By Name(cluster=T2 {"监测项描述:输出"="", "连接方式"=enum."串口", "端口"="", "IP address:"="", "Port:"="", "站号"=19200, "传感器型号"="", "波特率"=19200, "data bits"=8, "停止位"=10, "奇偶校验"=0} ("输出簇"), "监测项描述:输出"=w328, "端口"=w322, "站号"=u64 1, "传感器型号"=w320, "波特率"=u64 115200, "停止位"=u16 10, "奇偶校验"=u16 0, "data bits"=u64 8, "连接方式"=enum16{"串口", "TCP"}."串口", "IP address:"=w314, "Port:"=w314) -> (w325:T2)
            n113 = call <userlib>:"Write Section Cluster__ogtk.vi"("section (optional)"=w328, "error in (no error)"=w326, "Section Formatted Cluster"=w325, "refnum"=w327) -> ("error out"=w323:errorcluster, "dup refnum"=w324:T1)  [unwired: 6 in]
          }
          frame True {
          }
        }
      }
    }
    frame "浮船" {
      w412 = enum16{"串口", "TCP"}[] [enum."串口", enum."串口", enum."TCP"] items=["串口", "TCP"]
      w415 = enum16{"PLC", "ZLAN", "ART"}[] [enum."ART", enum."ZLAN", enum."ZLAN", enum."ZLAN", enum."ZLAN", enum."ZLAN", enum."ZLAN"] items=["PLC", "ZLAN", "ART"]
      w416 = T6 [enum."AI4", enum."DI0", enum."DI1", enum."DI2", enum."DI4", enum."DO2", enum."DO3"] items=["AI0", "AI1", "AI2", "AI3", "AI4", "DI0", "DI1", "DI2", "DI3", "DI4", "DO0", "DO1", "DO2", "DO3", "DO4", "X0", "X1", "X2", "X3", "X4", "X5", "X6", "X7", "X8", "X9"]
      w417 = enum32{"禁用告警", "闭合告警", "断开告警"}[] [enum."闭合告警", enum."闭合告警", enum."闭合告警", enum."闭合告警", enum."闭合告警", enum."闭合告警", enum."闭合告警"] items=["禁用告警", "闭合告警", "断开告警"]
      n114 = case shown="\"无配置开机恢复\", 默认" w413 {
        tunnel: [w428 TRUE ("empty?")] -> w414
        frame "无配置开机恢复", Default {
          n115 = global read "断电保存全局变量.vi" "配置ItemNames"() -> (w429:string[][])
          n116 = Empty Array?(array=w429) -> (empty?=w428:bool)
        }
        frame "手动恢复" {
        }
      }
      n117 = for {
        tunnel: string[] ["温湿度监测", "漏水监测", "烟雾监测", "门禁开关监测", "门禁开关监测2", "冰箱监测", "排气扇监测"] -> [w480] mode=indexing
        tunnel: w426 -> [w484]
        tunnel: w425 -> [w483]
        tunnel: w416 -> [w479] mode=indexing
        tunnel: w417 -> [w478] mode=indexing
        tunnel: w415 -> [w477] mode=indexing
        tunnel: [w476] -> w424
        tunnel: [w475] -> w423
        tunnel: w413 -> [w473]
        n118 = call <userlib>:"Read Section Cluster__ogtk.vi"("section (optional)"=w480, "error in (no error)"=w483, "Section Formatted Cluster Type"=T3 {"监测项描述:输出"="烟雾监测", "端口"=enum."X8", "告警方式"=enum."闭合告警", "传感器型号"=enum."PLC"} ("簇1输入"), "refnum"=w484) -> ("error out"=w481:errorcluster, "all found?"=w471:bool, "dup refnum"=w482:T1)  [unwired: 3 in, 2 out]
        n119 = case shown="\"无配置开机恢复\", 默认" w473 {
          tunnel: [w485 FALSE] -> w472
          tunnel: w471 -> [w485 _]
          frame "无配置开机恢复", Default {
          }
          frame "手动恢复" {
          }
        }
        n120 = case shown="假" w472 {
          tunnel: w482 -> [w500 w554]
          tunnel: w481 -> [w499 w553]
          tunnel: w480 -> [w490 _]
          tunnel: w479 -> [w498 _]
          tunnel: w478 -> [w497 _]
          tunnel: w477 -> [w496 _]
          tunnel: [w495 w554] -> w476
          tunnel: [w494 w553] -> w475
          frame False {
            n121 = Bundle By Name(cluster=T5 {"监测项描述:输出"="", "端口"=enum."AI0", "告警方式"=enum."禁用告警", "传感器型号"=enum."PLC", "声光告警启用"=FALSE} ("簇1输出"), "监测项描述:输出"=w490, "端口"=w498, "告警方式"=w497, "传感器型号"=w496, "声光告警启用"=FALSE) -> (w491:T5)
            n122 = global read "断电保存全局变量.vi" "IO监测配置输入"() -> (w493:T7)
            n123 = global read "断电保存全局变量.vi" "监测设备配置"() -> (w489:T8)
            n124 = call <userlib>:"Write Section Cluster__ogtk.vi"("section (optional)"=w490, "error in (no error)"=w499, "Section Formatted Cluster"=w491, "refnum"=w500) -> ("error out"=w494:errorcluster, "dup refnum"=w495:T1)  [unwired: 6 in]
            n125 = case shown="\"冰箱监测\"" w490 {
              tunnel: w493 -> [w502 w506 w510 w516 w522 w528 w534 w540 w546 w552]
              tunnel: [w502 w506 w510 w515 w521 w527 w533 w539 w545 w551] -> w492
              tunnel: w491 -> [_ _ _ w514 w520 w526 w532 w538 w544 w550]
              tunnel: w489 -> [w501 w505 w509 w513 w518 w524 w531 w537 w543 w549]
              tunnel: [w501 w503 w508 w512 w519 w525 w530 w536 w542 w548] -> _
              frame "假", Default {
              }
              frame "市电监测" {
                n126 = Bundle By Name(cluster=w505, "市电监测"=TRUE) -> (w503:T8)
              }
              frame "空调监测" {
                n127 = Bundle By Name(cluster=w509, "空调监测"=TRUE) -> (w508:T8)
              }
              frame "漏水监测" {
                n128 = Bundle By Name(cluster=w516, "漏水监测配置"=w514) -> (w515:T7)
                n129 = Bundle By Name(cluster=w513, "漏水监测"=TRUE) -> (w512:T8)
              }
              frame "门禁开关监测" {
                n130 = Bundle By Name(cluster=w522, "门禁开关监测配置"=w520) -> (w521:T7)
                n131 = Bundle By Name(cluster=w518, "门禁开关监测"=TRUE) -> (w519:T8)
              }
              frame "门禁开关监测2" {
                n132 = Bundle By Name(cluster=w528, "门禁开关监测配置2"=w526) -> (w527:T7)
                n133 = Bundle By Name(cluster=w524, "门禁开关监测2"=TRUE ("门禁开关监测")) -> (w525:T8)
              }
              frame "温湿度监测" {
                n134 = Bundle By Name(cluster=w534, "温湿度监测配置"=w532) -> (w533:T7)
                n135 = Bundle By Name(cluster=w531, "温度湿度"=TRUE) -> (w530:T8)
              }
              frame "烟雾监测" {
                n136 = Bundle By Name(cluster=w540, "烟雾监测配置"=w538) -> (w539:T7)
                n137 = Bundle By Name(cluster=w537, "温度湿度"=TRUE) -> (w536:T8)
              }
              frame "冰箱监测" {
                n138 = Bundle By Name(cluster=w546, "冰箱监测配置"=w544) -> (w545:T7)
                n139 = Bundle By Name(cluster=w543, "冰箱监测"=TRUE ("市电监测")) -> (w542:T8)
              }
              frame "排气扇监测" {
                n140 = Bundle By Name(cluster=w552, "排气扇监测配置"=w550) -> (w551:T7)
                n141 = Bundle By Name(cluster=w549, "排气扇监测"=TRUE) -> (w548:T8)
              }
            }
            n142 = global write "断电保存全局变量.vi" "IO监测配置输入"(w492) -> ()
          }
          frame True {
          }
        }
      }
      n143 = case shown="真" w414 {
        frame False {
        }
        frame True {
          n144 = global write "断电保存全局变量.vi" "配置ItemNames"(string[][] [["1", "温湿度监测", "ZLAN", "IO连接", "端口:AI4 闭合告警 启用声光告警", "编辑", "删除"], ["2", "漏水监测", "ZLAN", "IO连接", "端口:DI0 闭合告警 启用声光告警", "编辑", "删除"], ["3", "烟雾监测", "ZLAN", "IO连接", "端口:DI1 闭合告警 启用声光告警", "编辑", "删除"], ["4", "门禁开关监测", "ZLAN", "IO连接", "端口:DI2 断开告警 启用声光告警", "编辑", "删除"], ["5", "门禁开关监测2", "ZLAN", "IO连接", "端口:DI4 启用声光告警", "编辑", "删除"], ["5", "冰箱监测", "ZLAN", "IO连接", "端口:DO2 闭合告警 启用声光告警", "编辑", "删除"], ["6", "排气扇监测", "ZLAN", "IO连接", "端口:DO3 闭合告警 启用声光告警", "编辑", "删除"], ["7", "蓄电池监测", "太阳能控制器-MPPT12", "串口连接", "端口:COM1 站号:1 波特率:115200", "编辑", "删除"], ["8", "蓄电池监测2", "太阳能控制器-MPPT24", "串口连接", "端口:COM1 站号:2 波特率:115200", "编辑", "删除"], ["9", "GPS监测", "GPS", "TCP连接", "IP:192.168.1.1 Port:5001 不启用声光告警", "编辑", "删除"]] ("配置ItemNames")) -> ()
        }
      }
      n145 = for {
        tunnel: w424 -> [w449]
        tunnel: w423 -> [w448]
        tunnel: string[] ["蓄电池监测", "蓄电池监测2", "GPS监测"] -> [w447] mode=indexing
        tunnel: [w444] -> w421
        tunnel: [w443] -> w420
        tunnel: string[] ["COM1", "COM1", ""] -> [w442] mode=indexing
        tunnel: string[] ["太阳能控制器-MPPT12", "太阳能控制器-MPPT24", "GPS"] -> [w441] mode=indexing
        tunnel: w413 -> [w439]
        tunnel: w412 -> [w434] mode=indexing
        tunnel: string[] ["", "", "192.168.1.1"] -> [w433] mode=indexing
        tunnel: string[] ["", "", "5001"] -> [w432] mode=indexing
        i -> [w436]
        n146 = call <userlib>:"Read Section Cluster__ogtk.vi"("section (optional)"=w447, "error in (no error)"=w448, "Section Formatted Cluster Type"=T2 {"监测项描述:输出"="", "连接方式"=enum."串口", "端口"="", "IP address:"="", "Port:"="", "站号"=19200, "传感器型号"="", "波特率"=19200, "data bits"=8, "停止位"=10, "奇偶校验"=0} ("输出簇"), "refnum"=w449) -> ("error out"=w445:errorcluster, "all found?"=w438:bool, "dup refnum"=w446:T1)  [unwired: 3 in, 2 out]
        n147 = Increment(x=w436) -> (x+1=w435:i32)
        n148 = case shown="\"手动恢复\"" w439 {
          tunnel: [w450 FALSE] -> w437
          tunnel: w438 -> [w450 _]
          frame "无配置开机恢复", Default {
          }
          frame "手动恢复" {
          }
        }
        n149 = case shown="假" w437 {
          tunnel: w447 -> [w467 _]
          tunnel: w446 -> [w466 w470]
          tunnel: w445 -> [w465 w469]
          tunnel: [w463 w470] -> w444
          tunnel: [w462 w469] -> w443
          tunnel: w442 -> [w461 _]
          tunnel: w441 -> [w460 _]
          tunnel: w435 -> [w455 _]
          tunnel: w434 -> [w454 _]
          tunnel: w433 -> [w453 _]
          tunnel: w432 -> [w452 _]
          frame False {
            n150 = Bundle By Name(cluster=T2 {"监测项描述:输出"="", "连接方式"=enum."串口", "端口"="", "IP address:"="", "Port:"="", "站号"=19200, "传感器型号"="", "波特率"=19200, "data bits"=8, "停止位"=10, "奇偶校验"=0} ("输出簇"), "监测项描述:输出"=w467, "端口"=w461, "站号"=w455, "传感器型号"=w460, "波特率"=u64 115200, "停止位"=u16 10, "奇偶校验"=u16 0, "data bits"=u64 8, "连接方式"=w454, "IP address:"=w453, "Port:"=w452) -> (w464:T2)
            n151 = call <userlib>:"Write Section Cluster__ogtk.vi"("section (optional)"=w467, "error in (no error)"=w465, "Section Formatted Cluster"=w464, "refnum"=w466) -> ("error out"=w462:errorcluster, "dup refnum"=w463:T1)  [unwired: 6 in]
          }
          frame True {
          }
        }
      }
    }
  }
  n152 = call <vilib>:"Close Config Data.vi"("error in (no error)"=w8, "refnum"=w9) -> ("error out"=w2:errorcluster)  [unwired: 8 in, 1 out]
  n153 = call "save.vi"("error in (no error)"=w2) -> ("error out"=→"error out":errorcluster)  [unwired: 10 in]
